vi "Get Number 6 Digit 2.vi"(11 "Array":string[][](array[string])) -> (2 "String":string, 3 "Result":string)   [LabVIEW 2019, in "Day 8.lvlib"]
uses:
  Day 8.lvlib
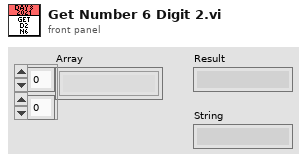
[diagram p1: front panel]
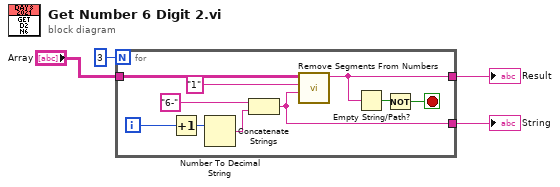
[diagram p0: block diagram]
diagram:
  n1 = for {
    N: 3 -> [_]
    tunnel: "Array" -> [w14]
    tunnel: [w8] -> w1
    tunnel: [w5] -> w4
    i -> [w9]
    stop <- w6 stop-if-true
    n2 = Increment(x=w9) -> (x+1=w10:i32)
    n3 = Number To Decimal String(number=w10) -> (decimal integer string=w11:string)  [unwired: 1 in]
    n4 = Concatenate Strings("6-" ("Pattern For Number Of Letters A"), w11) -> (w5:string)
    n5 = call "Remove Segments From Numbers.vi"("Pattern For Letter Of Letters B"=w5, "Pattern For Number Of Letters A"="1", "Array"=w14) -> ("Result"=w8:string)  [unwired: 8 in]
    n6 = Empty String/Path?(string/path=w8) -> (empty?=w7:bool)
    n7 = Not(x=w7) -> (.not. x?=w6:bool)
  }
  "String" <- w4
  "Result" <- w1
